vi "Cam H.vi"() -> ()   [LabVIEW 2016]
panel:
  out "Cam H":dbl
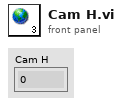
[diagram p1: front panel]
diagram:
